vi "GetJibSailPos.vi"(8 "error in (no error)":errorcluster, 11 "AbstractSail in":refnum<class "AbstractSail.lvclass">) -> (0 "error out":errorcluster, 2 "MainSailPos":dbl, 3 "AbstractSail out":refnum<class "AbstractSail.lvclass">)   [LabVIEW 2011, in "AbstractSail.lvclass"]
uses:
  AbstractSail.lvclass
  AbstractSail.lvclass/AbstractSail.ctl
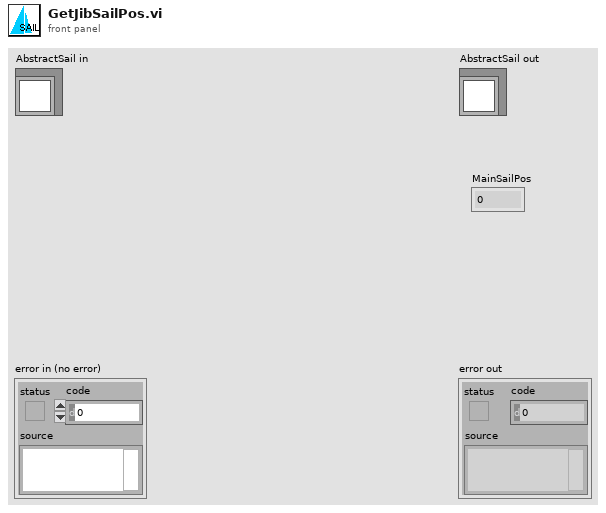
[diagram p1: front panel]
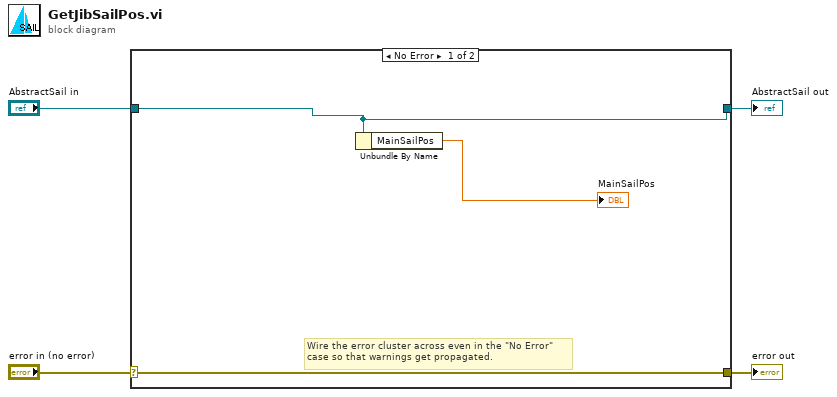
[diagram p0: block diagram]
diagram:
  n1 = case shown="No Error" "error in (no error)" {
    selector: "error in (no error)" -> [w7 w9]
    tunnel: [w7 w9] -> w3
    tunnel: [w6 w8] -> w1
    tunnel: "AbstractSail in" -> [w6 w8]
    frame No Error {
      # "Wire the error cluster across even in the \"No Error\"\ncase so that warnings get propagated."
      n2 = Unbundle By Name(w6) -> ("MainSailPos"=→"MainSailPos":dbl)
    }
    frame Error {
    }
  }
  "error out" <- w3
  "AbstractSail out" <- w1
